vi "Modbus Convert Temperature.vi"(8 "error in":errorcluster, 11 "PLC Value":u16) -> (0 "error out":errorcluster, 3 "Converted Value":dbl)   [LabVIEW 2020, in "Modbus.lvlib"]
uses:
  Modbus.lvlib
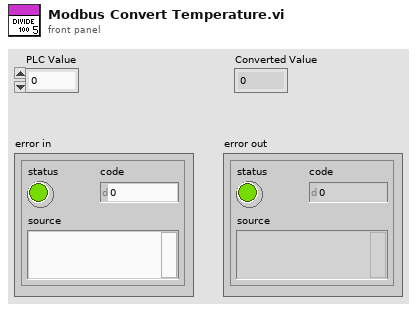
[diagram p1: front panel]
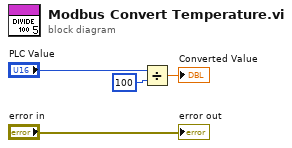
[diagram p0: block diagram]
diagram:
  n1 = Divide(x="PLC Value", y=u16 100) -> (x/y=→"Converted Value":dbl)
  "error out" <- "error in"
